vi "Get Loaded Robot Program.vi"(8 "error in (no error)":errorcluster, 11 "UR5 Robot in":refnum<class "UR5 Robot.lvclass">) -> (0 "error out":errorcluster, 3 "UR5 Robot out":refnum<class "UR5 Robot.lvclass">)   [LabVIEW 2018, in "UR5 Robot.lvlib" / "UR5 Robot.lvclass"]
uses:
  UR5 Robot.lvclass
  UR5 Robot.lvclass/UR5 Robot.ctl
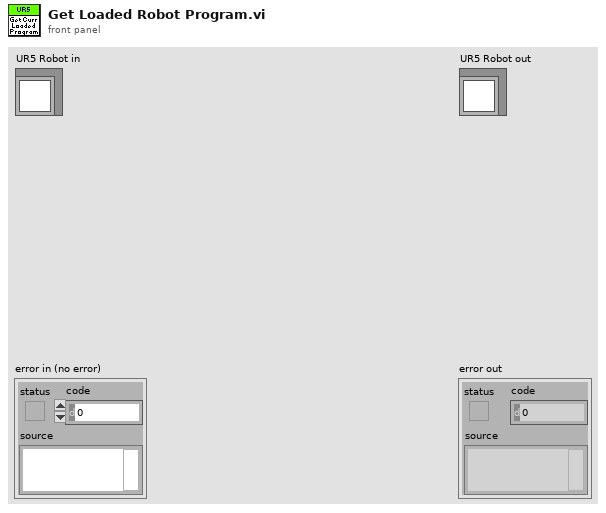
[diagram p1: front panel]
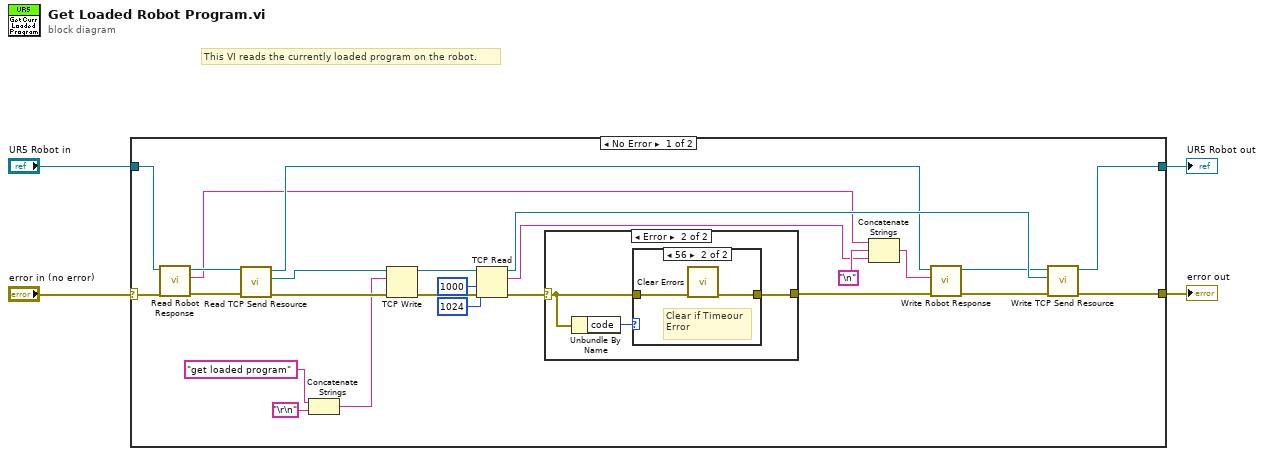
[diagram p0: block diagram]
diagram:
  # "This VI reads the currently loaded program on the robot."
  n1 = case shown="No Error" "error in (no error)" {
    selector: "error in (no error)" -> [w19 w38]
    tunnel: [w22 w38] -> w3
    tunnel: [w20 w37] -> w1
    tunnel: "UR5 Robot in" -> [w17 w37]
    frame No Error {
      n2 = call "Read Robot Response.vi"("error in (no error)"=w19, "UR5 Robot in"=w17) -> ("error out"=w18:errorcluster, "Robot Response"=w11:string, "UR5 Robot out"=w16:refnum<class "UR5 Robot.lvclass">)  [unwired: 7 in]
      n3 = call "Read TCP Send Resource.vi"("error in (no error)"=w18, "UR5 Robot in"=w16) -> ("error out"=w23:errorcluster, "TCP Send Resource"=w24:refnum<k5>, "UR5 Robot out"=w13:refnum<class "UR5 Robot.lvclass">)  [unwired: 7 in]
      n4 = Concatenate Strings("get loaded program", "\r\n") -> (w5:string)
      n5 = TCP Write(connection ID=w24, data in=w5, error in (no error)=w23) -> (connection ID out=w28:refnum<k5>, error out=w27:errorcluster)  [unwired: 1 in, 1 out]
      n6 = TCP Read(connection ID=w28, bytes to read=1024, error in (no error)=w27, 9:1000 ("timeout ms (25000)")) -> (connection ID out=w21:refnum<k5>, data out=w9:string, error out=w29:errorcluster)  [unwired: 1 in]
      n7 = case shown="Error" w29 {
        selector: w29 -> [w30 w32]
        tunnel: [w30 w31] -> w15
        frame No Error {
        }
        frame Error {
          n8 = Unbundle By Name(w32) -> ("code"=w33:i32)
          n9 = case shown="56" w33 {
            tunnel: w32 -> [w34 w36]
            tunnel: [w34 w35] -> w31
            frame 0, Default {
            }
            frame 56 {
              # "Clear if Timeour\nError"
              n10 = call <vilib>:"Clear Errors.vi"("error in (no error)"=w36) -> ("error out"=w35:errorcluster)  [unwired: 5 in, 1 out]
            }
          }
        }
      }
      n11 = Concatenate Strings(w11, "\n", w9) -> (w8:string)
      n12 = call "Write Robot Response.vi"("error in (no error)"=w15, "Robot Response"=w8, "UR5 Robot in"=w13) -> ("error out"=w14:errorcluster, "UR5 Robot out"=w12:refnum<class "UR5 Robot.lvclass">)  [unwired: 7 in]
      n13 = call "Write TCP Send Resource.vi"("error in (no error)"=w14, "TCP Send Resource"=w21, "UR5 Robot in"=w12) -> ("error out"=w22:errorcluster, "UR5 Robot out"=w20:refnum<class "UR5 Robot.lvclass">)  [unwired: 7 in]
    }
    frame Error {
    }
  }
  "error out" <- w3
  "UR5 Robot out" <- w1
